vi "Total SV.vi"(11 "All Lines":string[](array[string])) -> (3 "Final Output":string[](array[string]))   [LabVIEW 2025]
panel:
  out "String 2":string
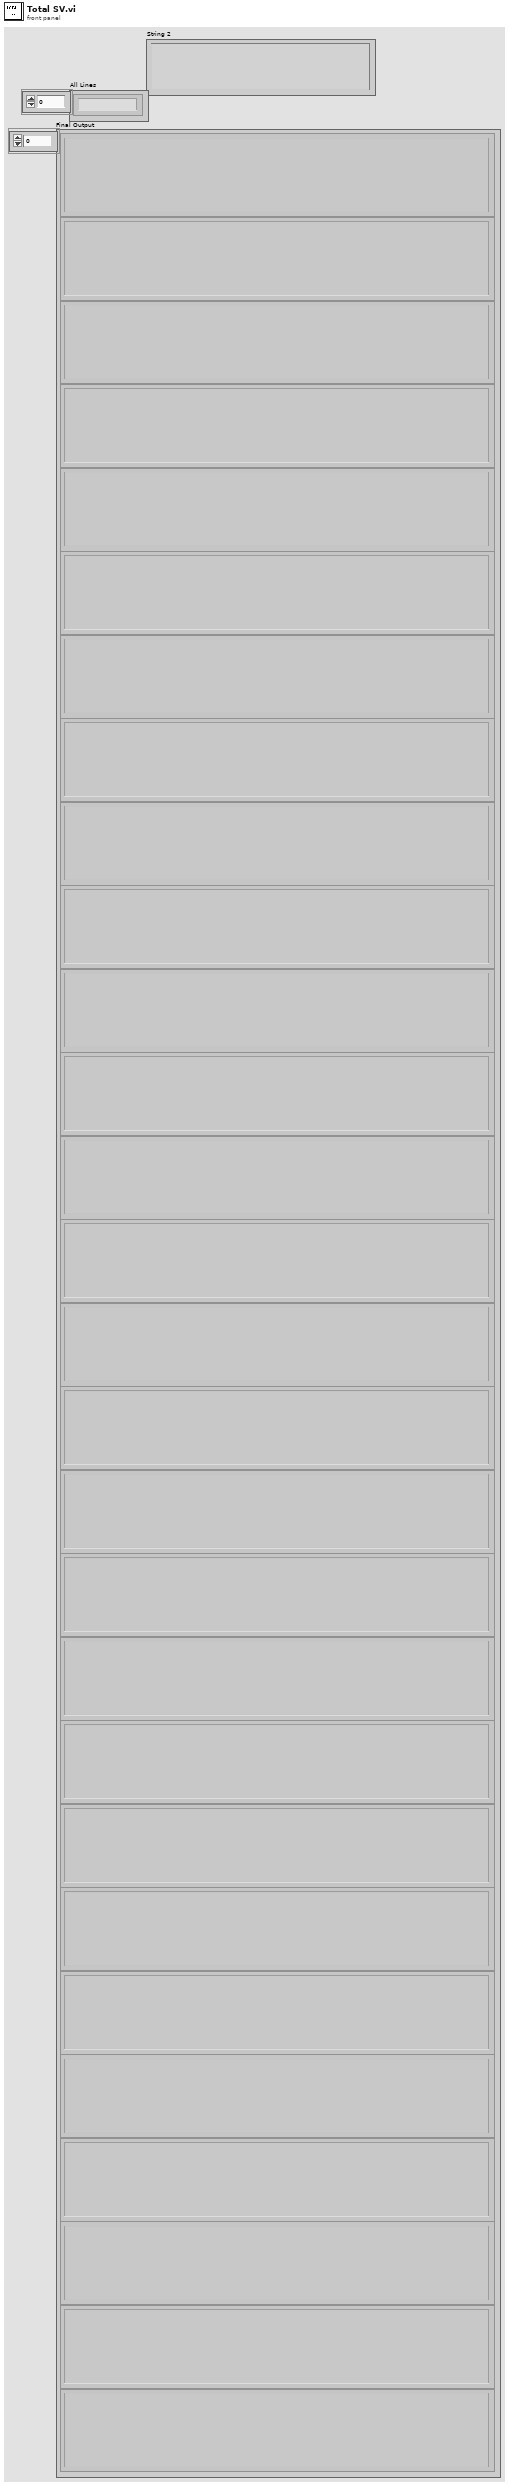
[diagram p1: front panel]
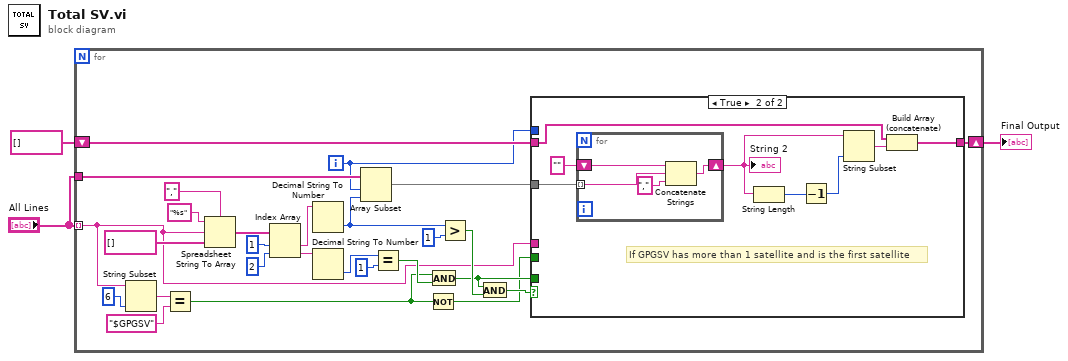
[diagram p0: block diagram]
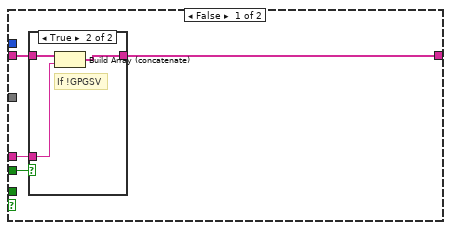
[diagram p2: hidden frame]
diagram:
  n1 = for {
    tunnel: "All Lines" -> [w4] mode=indexing
    shift-right: [w12] -> w3
    shift-left: string[] [] -> [w13]
    tunnel: "All Lines" -> [w11]
    i -> [w7]
    n2 = String Subset(string=w4, length (rest)=6 ("length (rest)")) -> (substring=w29:string)  [unwired: 1 in]
    n3 = Equal?(x=w29, y="$GPGSV") -> (x = y?=w6:bool)
    n4 = Spreadsheet String To Array(delimiter (Tab)=",", format string="%s" ("spreadsheet string"), spreadsheet string=w4, array type (2D Dbl)=string[] []) -> (array=w24:string[])
    n5 = Index Array(array=w24, index #1=1 ("disabled index (col)"), index #2=2 ("index")) -> (element #1=w22:string, element #2=w18:string)
    n6 = Decimal String To Number(string=w22) -> (number=w14:i32)  [unwired: 2 in, 1 out]
    n7 = Decimal String To Number(string=w18) -> (number=w17:i32)  [unwired: 2 in, 1 out]
    n8 = Array Subset(array=w11, index=w7, length=w14) -> (w20:string[])
    n9 = Equal?(x=w17, y=1) -> (x = y?=w10:bool)
    n10 = Not(x=w6) -> (.not. x?=w5:bool)
    n11 = And(x=w6, y=w10) -> (x .and. y?=w8:bool)
    n12 = Greater?(x=w14, y=1) -> (0:w9:bool)
    n13 = And(x=w8, y=w9) -> (x .and. y?=w15:bool)
    n14 = case shown="True" w15 {
      tunnel: w20 -> [_ w45]
      tunnel: [w34 w39] -> w12
      tunnel: w13 -> [w33 w40]
      tunnel: w4 -> [w32 _]
      tunnel: w8 -> [_ _]
      tunnel: w7 -> [_ _]
      tunnel: w5 -> [w31 _]
      frame False {
        n15 = case shown="True" w31 {
          tunnel: w33 -> [w35 w38]
          tunnel: [w35 w37] -> w34
          tunnel: w32 -> [_ w36]
          frame False {
          }
          frame True {
            # "If !GPGSV"
            n16 = Build Array (concatenate)(w38, w36) -> (w37:string[])
          }
        }
      }
      frame True {
        # "If GPGSV has more than 1 satellite and is the first satellite"
        n17 = for {
          tunnel: w45 -> [w50] mode=indexing
          shift-right: [w49] -> w42
          shift-left: "" -> [w48]
          n18 = Concatenate Strings(w48, w50, "," ("string")) -> (w49:string)
        }
        "String 2" <- w42
        n19 = String Length(string=w42) -> (length=w43:i32)
        n20 = Decrement(x=w43) -> (x-1=w44:i32)
        n21 = String Subset(string=w42, length (rest)=w44) -> (substring=w41:string)  [unwired: 1 in]
        n22 = Build Array (concatenate)(w40, w41) -> (w39:string[])
      }
    }
  }
  "Final Output" <- w3
